vi "List Sensor File.vi"(8 "error in (no error)":errorcluster, 11 "Main Model in":refnum<class "Main Model.lvclass">) -> (0 "error out":errorcluster, 3 "Main Model out":refnum<class "Main Model.lvclass">)   [LabVIEW 2013, in "Main Model.lvlib" / "Main Model.lvclass"]
uses:
  Main Model.lvclass
  Main Model.lvclass/Main Model.ctl
  Common/File IO/File IO.lvlib
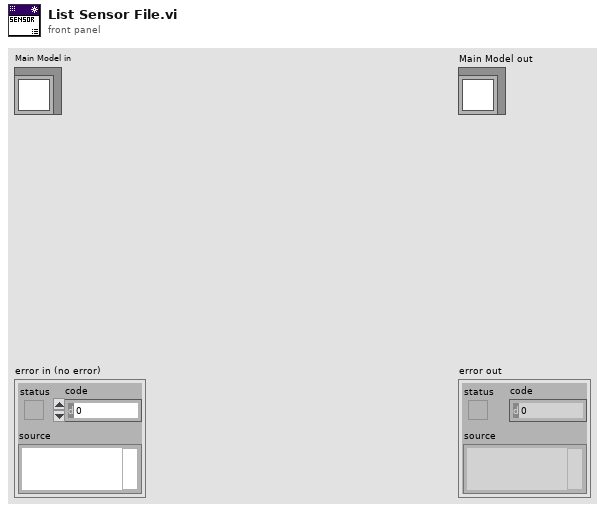
[diagram p1: front panel]
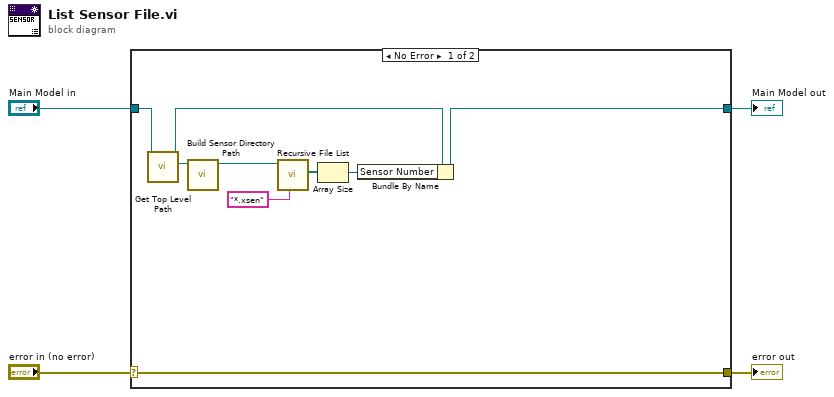
[diagram p0: block diagram]
diagram:
  n1 = case shown="No Error" "error in (no error)" {
    selector: "error in (no error)" -> [w13 w15]
    tunnel: [w13 w15] -> w3
    tunnel: [w5 w14] -> w1
    tunnel: "Main Model in" -> [w12 w14]
    frame No Error {
      n2 = call-dynamic "Get Top Level Path.vi"("Abstract Model in"=w12) -> ("Top Level Path"=w11:path, "Abstract Model out"=w7:refnum<class "Main Model.lvclass">)  [unwired: 8 in, 1 out]
      n3 = call "Build Sensor Directory Path.vi"("Top Level Path"=w11) -> ("Sensor Directory Path"=w10:path)  [unwired: 10 in]
      n4 = call <vilib>:"Recursive File List.vi"("pattern"="*.xsen", "Folder Path"=w10) -> ("All Files in Dir"=w8:path[])  [unwired: 5 in, 4 out]
      n5 = Array Size(array=w8) -> (size(s)=w6:i32)
      n6 = Bundle By Name(cluster=w7, "Sensor Number"=w6) -> (w5:refnum<class "Main Model.lvclass">)
    }
    frame Error {
    }
  }
  "error out" <- w3
  "Main Model out" <- w1
